vi "Write Car Wash Controller.vi"(8 "error in (no error)":errorcluster, 10 "Architecture.lvlib:Queue.lvclass":refnum<class "Queue.lvclass">, 11 "Entry Console in":refnum<class "Entry Console.lvclass">) -> (0 "error out":errorcluster, 3 "Entry Console out":refnum<class "Entry Console.lvclass">)   [LabVIEW 2016, in "Entry Console.lvlib" / "Entry Console.lvclass"]
uses:
  Entry Console.lvclass
  Queue/Queue.lvclass
  Entry Console.lvclass/Entry Console.ctl
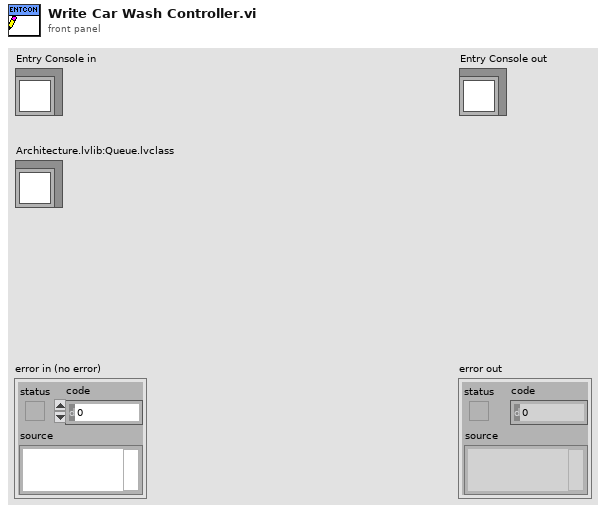
[diagram p1: front panel]
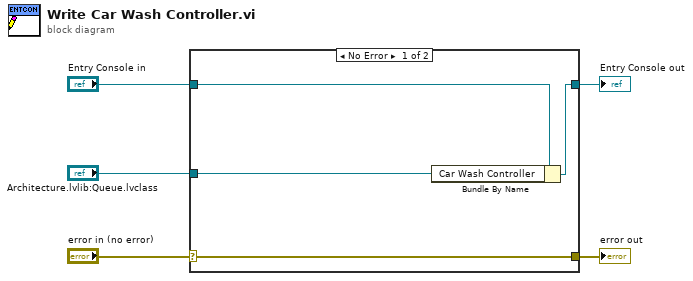
[diagram p0: block diagram]
diagram:
  n1 = case shown="No Error" "error in (no error)" {
    selector: "error in (no error)" -> [w9 w10]
    tunnel: [w9 w10] -> w4
    tunnel: [w7 w11] -> w2
    tunnel: "Entry Console in" -> [w8 w11]
    tunnel: "Architecture.lvlib:Queue.lvclass" -> [w6 _]
    frame No Error {
      n2 = Bundle By Name(cluster=w8, "Car Wash Controller"=w6) -> (w7:refnum<class "Entry Console.lvclass">)
    }
    frame Error {
    }
  }
  "error out" <- w4
  "Entry Console out" <- w2
